vi "checkMinMaxScale.vi"(0 "Camera in":refnum<class "Camera.lvclass">, 5 "data_format":T1(ring)=enum."Mono16", 11 "error in (no error)":errorcluster) -> (4 "Camera out":refnum<class "Camera.lvclass">, 6 "needsUpdate":bool, 15 "error out":errorcluster)   [LabVIEW 2019, in "Camera.lvclass"]
doc: "Checks if the minimum and maximum scale of the convert settings need to be adapted\nand updates them if necessary\n\nThis is needed to ensure that no \"color overflow\" occurs, which might produce strange color artifacts"
uses:
  Camera.lvclass
  Camera.lvclass/Camera.ctl
  pco.convert/Convert.lvlib
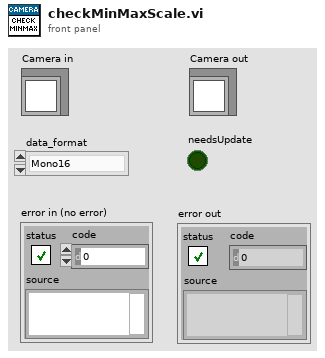
[diagram p1: front panel]
types:
  T1 = enum16{"Undefined", "Mono8", "Mono16", "BGRA8", "RGBA8", "BGRA16", "RGBA16", "CompressedMono8"}
  T2 = map{enum16{"Undefined", "Mono8", "Mono16", "BGRA8", "RGBA8", "BGRA16", "RGBA16", "CompressedMono8"}, cluster{"sharpen":bool, "adaptive_sharpen":bool, "flip_vertical":bool, "auto_minmax":bool, "add_conv_flags":u32, "min_limit":u16, "max_limit":u16, "gamma":dbl, "contrast":i32, "pco_debayer_algorithm":bool, "color_temperature":i32, "color_saturation":i32, "color_vibrance":i32, "color_tint":i32, "lut_file":path}}
  T3 = cluster{"sharpen":bool, "adaptive_sharpen":bool, "flip_vertical":bool, "auto_minmax":bool, "add_conv_flags":u32, "min_limit":u16, "max_limit":u16, "gamma":dbl, "contrast":i32, "pco_debayer_algorithm":bool, "color_temperature":i32, "color_saturation":i32, "color_vibrance":i32, "color_tint":i32, "lut_file":path}
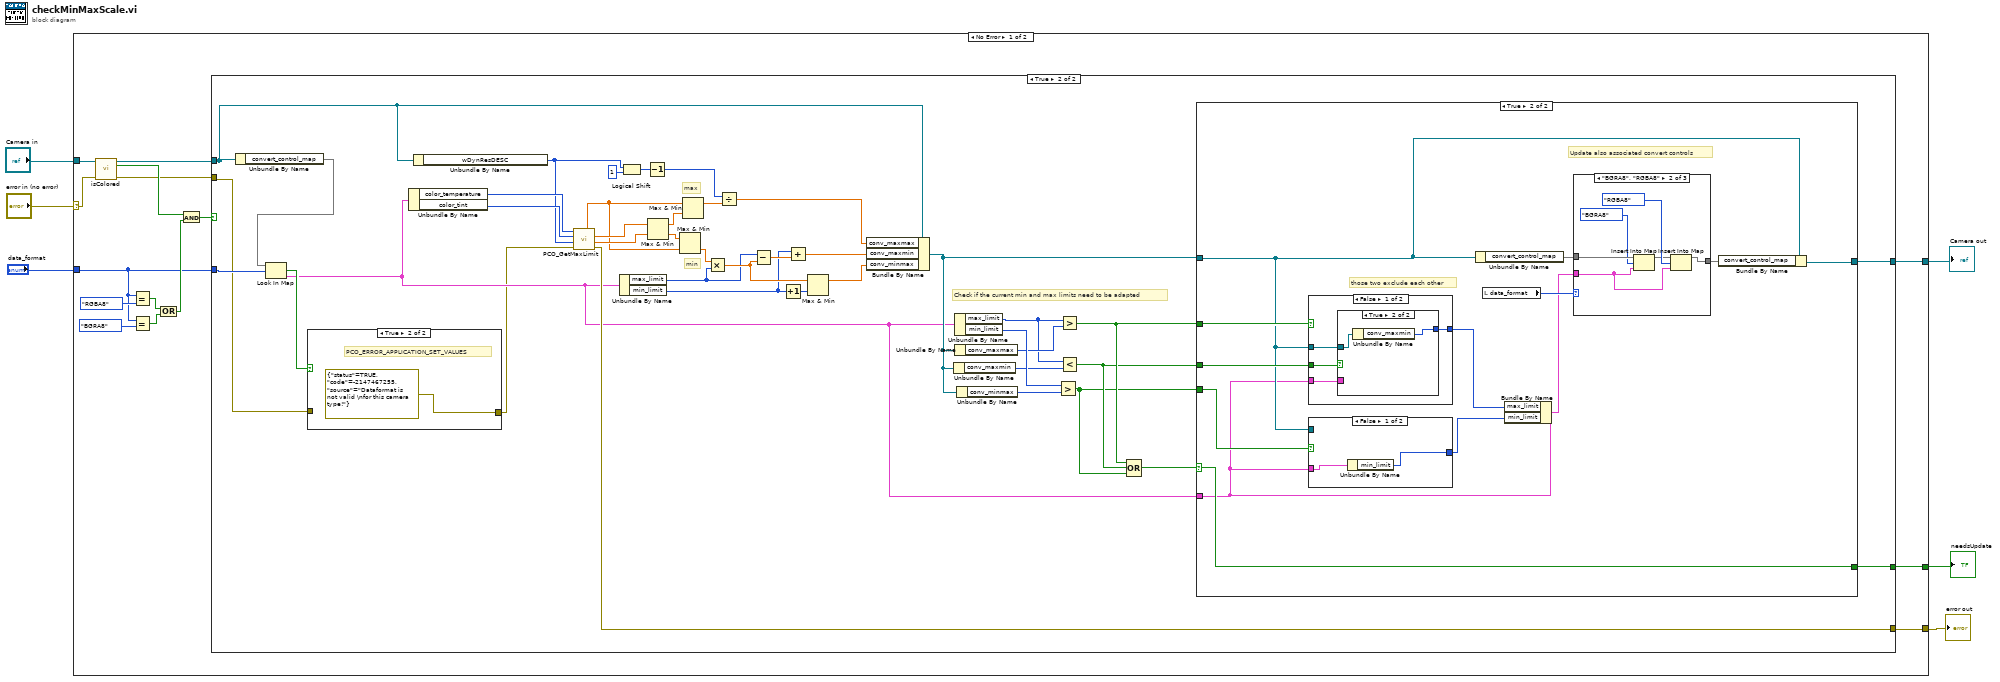
[diagram p0: block diagram]
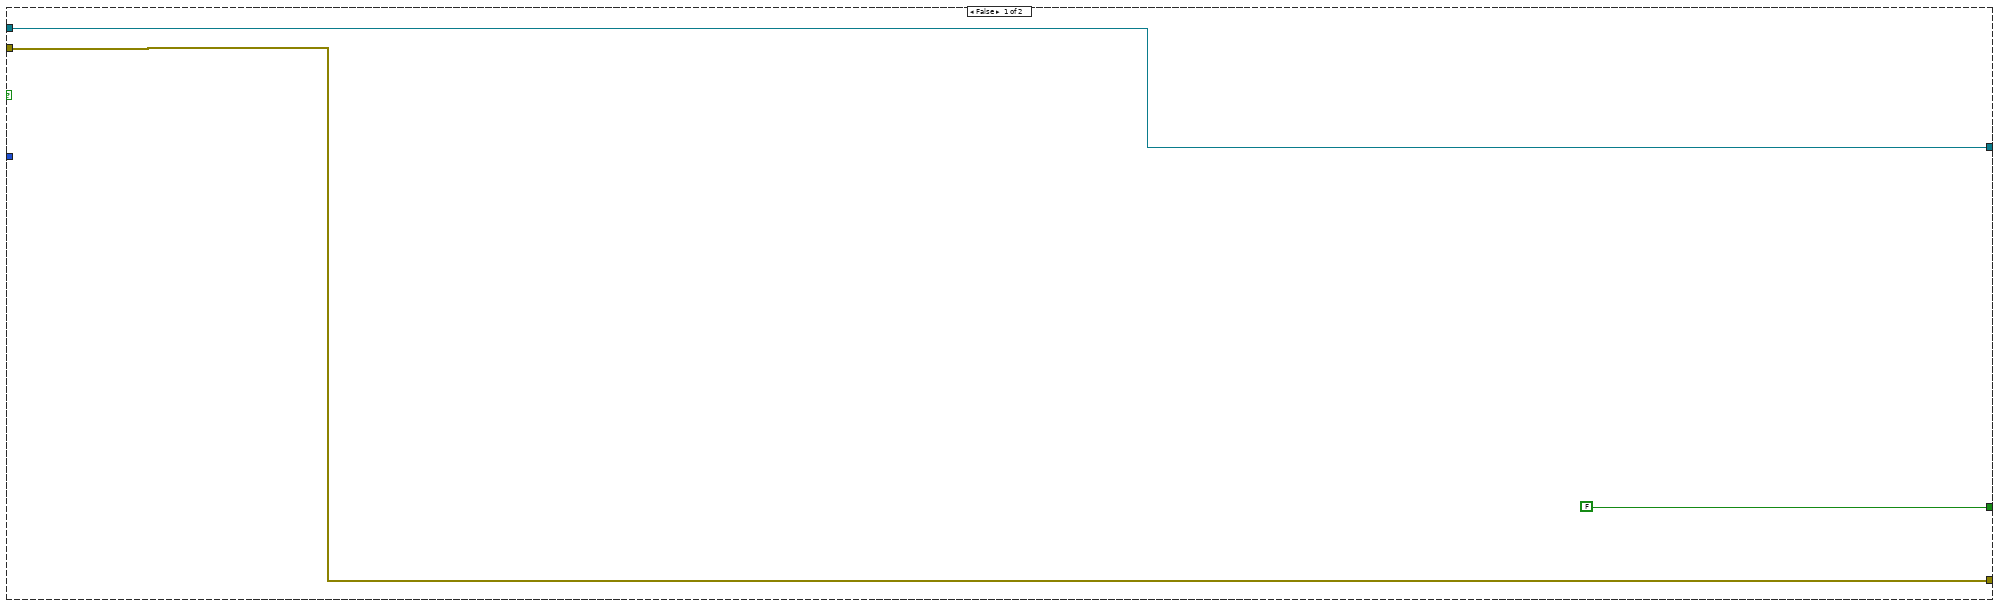
[diagram p2: hidden frame]
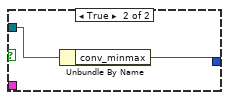
[diagram p5: hidden frame]
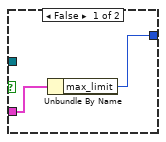
[diagram p6: hidden frame]
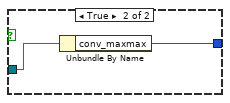
[diagram p7: hidden frame]
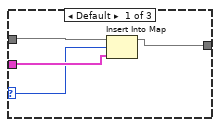
[diagram p8: hidden frame]
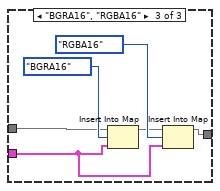
[diagram p9: hidden frame]
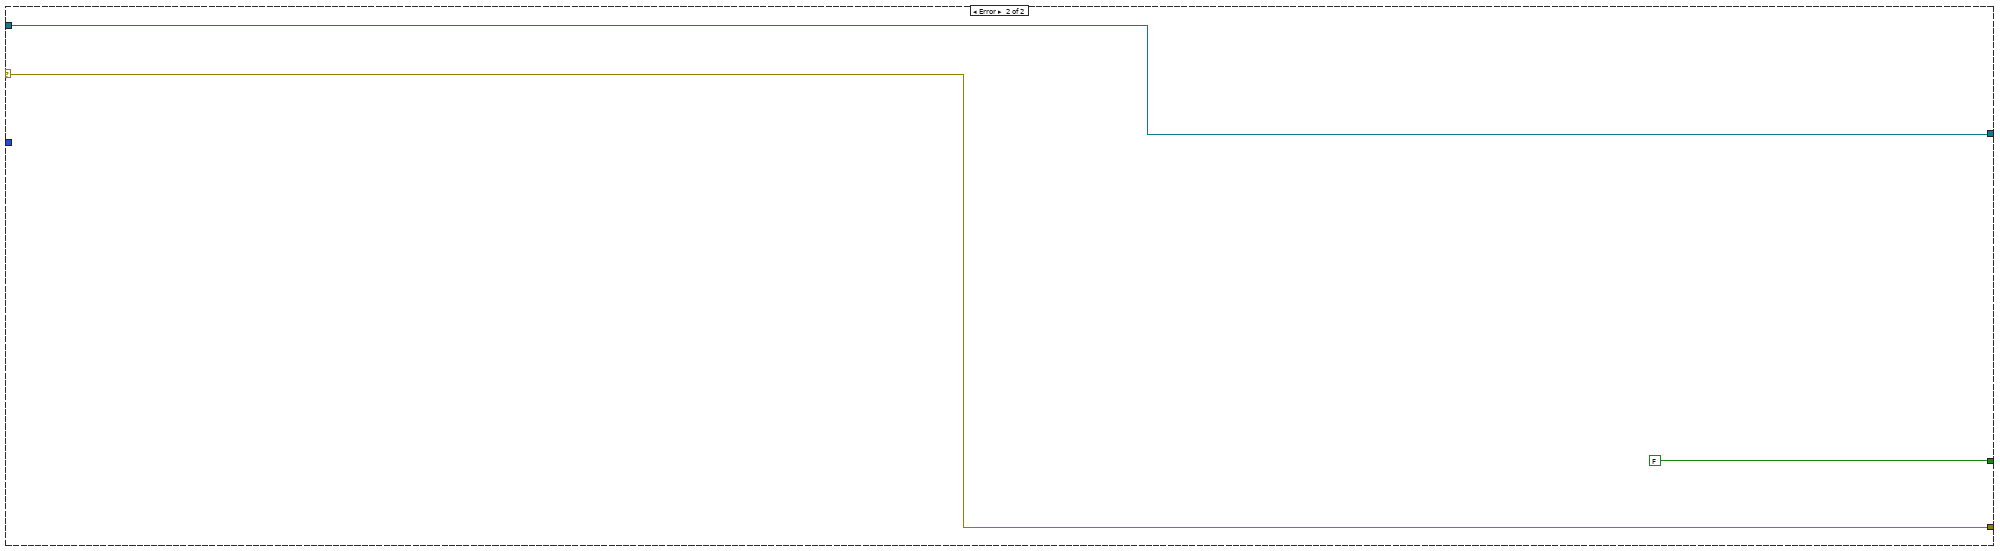
[diagram p10: hidden frame]
diagram:
  n1 = case shown="No Error" "error in (no error)" {
    selector: "error in (no error)" -> [w14 w115]
    tunnel: "Camera in" -> [w21 w113]
    tunnel: "data_format" -> [w11 _]
    tunnel: [w10 w115] -> w2
    tunnel: [w9 w113] -> w1
    tunnel: [w8 FALSE] -> w3
    frame No Error {
      n2 = call-dynamic "isColored.vi"("Camera in"=w21, "error in (no error)"=w14) -> ("Camera out"=w15:refnum<class "Camera.lvclass">, "colored"=w17:bool, "error out"=w13:errorcluster)  [unwired: 11 in]
      n3 = Equal?(x=w11, y=T1."RGBA8" ("data_format")) -> (x = y?=w19:bool)
      n4 = Equal?(x=w11, y=T1."BGRA8" ("data_format")) -> (x = y?=w18:bool)
      n5 = Compound Arithmetic op=OR(w19, w18) -> (w16:bool)
      n6 = Compound Arithmetic op=AND(w17, w16) -> (w12:bool)
      n7 = case shown="True" w12 {
        tunnel: w15 -> [w22 w26]
        tunnel: w13 -> [w23 w27]
        tunnel: w11 -> [_ w29]
        tunnel: [w23 w40] -> w10
        tunnel: [w22 w39] -> w9
        tunnel: [FALSE w38] -> w8
        frame False {
        }
        frame True {
          # "Check if the current min and max limits need to be adapted"
          # "min"
          # "max"
          n8 = Unbundle By Name(w26) -> ("convert_control_map"=w30:T2)
          n9 = Look In Map(map=w30, key=w29) -> (key not found?=w31:bool, value=w28:T3)  [unwired: 1 in]
          n10 = case shown="True" w31 {
            tunnel: w27 -> [w66 _]
            tunnel: [w66 errorcluster {"status"=TRUE, "code"=-2147467255, "source"="Dataformat is not valid \nfor this camera type!"} ("error IO")] -> w25
            frame False {
            }
            frame True {
              # "PCO_ERROR_APPLICATION_SET_VALUES"
            }
          }
          n11 = Unbundle By Name(w28) -> ("color_temperature"=w65:i32, "color_tint"=w64:i32)
          n12 = Unbundle By Name(w26) -> ("wDynResDESC"=w57:u16)
          n13 = call "PCO_GetMaxLimit.vi"("error in (no error)"=w25, "output_bits"=w57, "tint"=w64, "temp"=w65) -> ("error out"=w40:errorcluster, "g_max"=w63:sgl, "r_max"=w62:sgl, "b_max"=w59:sgl)  [unwired: 3 in, 1 out]
          n14 = Unbundle By Name(w28) -> ("max_limit"=w46:u16, "min_limit"=w45:u16)
          n15 = Logical Shift(y=w57, x=u32 1) -> (x << y=w56:u32)
          n16 = Decrement(x=w56) -> (x-1=w55:u32)
          n17 = Max & Min(x=w62, y=w63) -> (max(x,y)=w61:sgl, min(x,y)=w60:sgl)
          n18 = Max & Min(x=w60, y=w59) -> (min(x,y)=w52:sgl)  [unwired: 1 out]
          n19 = Max & Min(x=w59, y=w61) -> (max(x,y)=w54:sgl)  [unwired: 1 out]
          n20 = Multiply(x=w52, y=w46) -> (x*y=w47:sgl)
          n21 = Divide(x=w55, y=w54) -> (x/y=w53:sgl)
          n22 = Subtract(x=w46, y=w47) -> (x-y=w49:sgl)
          n23 = Increment(x=w45) -> (x+1=w51:u16)
          n24 = Add(x=w45, y=w49) -> (x+y=w48:sgl)
          n25 = Max & Min(x=w47, y=w51) -> (max(x,y)=w50:sgl)  [unwired: 1 out]
          n26 = Bundle By Name(cluster=w26, "conv_maxmax"=w53, "conv_maxmin"=w48, "conv_minmax"=w50) -> (w32:refnum<class "Camera.lvclass">)
          n27 = Unbundle By Name(w32) -> ("conv_maxmin"=w36:i32)
          n28 = Unbundle By Name(w28) -> ("max_limit"=w37:u16, "min_limit"=w44:u16)
          n29 = Unbundle By Name(w32) -> ("conv_maxmax"=w43:i32)
          n30 = Unbundle By Name(w32) -> ("conv_minmax"=w42:i32)
          n31 = Greater?(x=w44, y=w42) -> (0:w33:bool)
          n32 = Greater?(x=w37, y=w43) -> (0:w35:bool)
          n33 = Less?(x=w37, y=w36) -> (x < y?=w34:bool)
          n34 = Compound Arithmetic op=OR(w35, w34, w33) -> (w41:bool)
          n35 = case shown="True" w41 {
            selector: w41 -> [w69 w82]
            tunnel: w28 -> [_ w71]
            tunnel: [w69 w82] -> w38
            tunnel: [w68 w77] -> w39
            tunnel: w35 -> [_ w76]
            tunnel: w34 -> [_ w75]
            tunnel: w33 -> [_ w73]
            tunnel: w32 -> [w68 w72]
            frame False {
            }
            frame True {
              # "those two exclude each other"
              # "Update also associated convert controls"
              n36 = case shown="False" w76 {
                tunnel: w75 -> [w90 _]
                tunnel: [w89 w96] -> w74
                tunnel: w72 -> [w88 w95]
                tunnel: w71 -> [w87 _]
                frame False {
                  n37 = case shown="True" w90 {
                    tunnel: w88 -> [_ w94]
                    tunnel: [w92 w93] -> w89
                    tunnel: w87 -> [w91 _]
                    frame False {
                      n38 = Unbundle By Name(w91) -> ("max_limit"=w92:u16)
                    }
                    frame True {
                      n39 = Unbundle By Name(w94) -> ("conv_maxmin"=w93:i32)
                    }
                  }
                }
                frame True {
                  n40 = Unbundle By Name(w95) -> ("conv_maxmax"=w96:i32)
                }
              }
              n41 = case shown="False" w73 {
                tunnel: w72 -> [_ w86]
                tunnel: w71 -> [w84 _]
                tunnel: [w83 w85] -> w70
                frame False {
                  n42 = Unbundle By Name(w84) -> ("min_limit"=w83:u16)
                }
                frame True {
                  n43 = Unbundle By Name(w86) -> ("conv_minmax"=w85:i32)
                }
              }
              n44 = Unbundle By Name(w72) -> ("convert_control_map"=w79:T2)
              n45 = local read "data_format"() -> (w80:T1)
              n46 = Bundle By Name(cluster=w71, "max_limit"=w74, "min_limit"=w70) -> (w78:T3)
              n47 = case shown="\"BGRA8\", \"RGBA8\"" w80 {
                selector: w80 -> [w98 _ _]
                tunnel: w79 -> [w99 w106 w108]
                tunnel: w78 -> [w100 w104 w107]
                tunnel: [w97 w101 w109] -> w81
                frame Default {
                  n48 = Insert Into Map(map in=w99, key=w98, value=w100) -> (map out=w97:T2)  [unwired: 2 out]
                }
                frame "BGRA8", "RGBA8" {
                  n49 = Insert Into Map(map in=w106, key=T1."BGRA8" ("data_format"), value=w104) -> (map out=w102:T2)  [unwired: 2 out]
                  n50 = Insert Into Map(map in=w102, key=T1."RGBA8" ("data_format"), value=w104) -> (map out=w101:T2)  [unwired: 2 out]
                }
                frame "BGRA16", "RGBA16" {
                  n51 = Insert Into Map(map in=w108, key=T1."BGRA16" ("data_format"), value=w107) -> (map out=w110:T2)  [unwired: 2 out]
                  n52 = Insert Into Map(map in=w110, key=T1."RGBA16" ("data_format"), value=w107) -> (map out=w109:T2)  [unwired: 2 out]
                }
              }
              n53 = Bundle By Name(cluster=w72, "convert_control_map"=w81) -> (w77:refnum<class "Camera.lvclass">)
            }
          }
        }
      }
    }
    frame Error {
    }
  }
  "error out" <- w2
  "Camera out" <- w1
  "needsUpdate" <- w3
